vi "DPO_7K_NextState_Autoscale.vi"(5 "Upper Threshold":dbl, 6 "ATI?":bool, 7 "Lower Threshold":dbl, 8 "Offset":dbl, 9 "Current Vertical Scale":dbl, 10 "Waveform Maximum Value":dbl, 11 "Waveform Minumum Value":dbl) -> (3 "Autoscale States":T1)   [LabVIEW 2020]
uses:
  DPO_7K_Autoscale_States.ctl
panel:
  out "Minimum":dbl
  out "Maximum":dbl
  out "Acquisition warning":bool
  out "Increase vertical scale":bool
  out "Decrease vertical scale":bool
  out "Change Offset":bool
  out "Valid Acquisition, Exit":bool
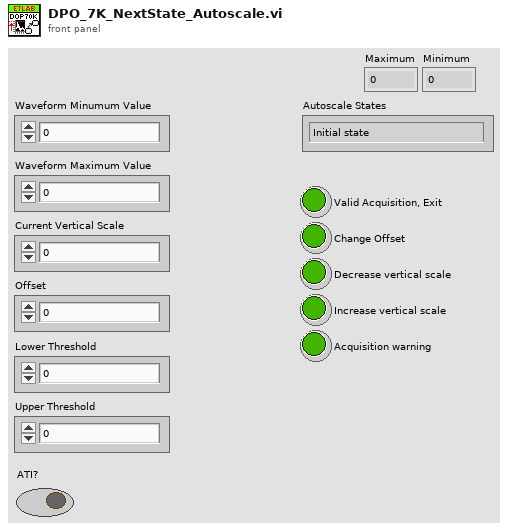
[diagram p1: front panel]
types:
  T1 = typedef "DPO_7K_Autoscale_States.ctl" = enum16{"Initial state", "Change offset", "Increase scale", "Decrease scale", "Acquisition warning", "General error", "Exit"}
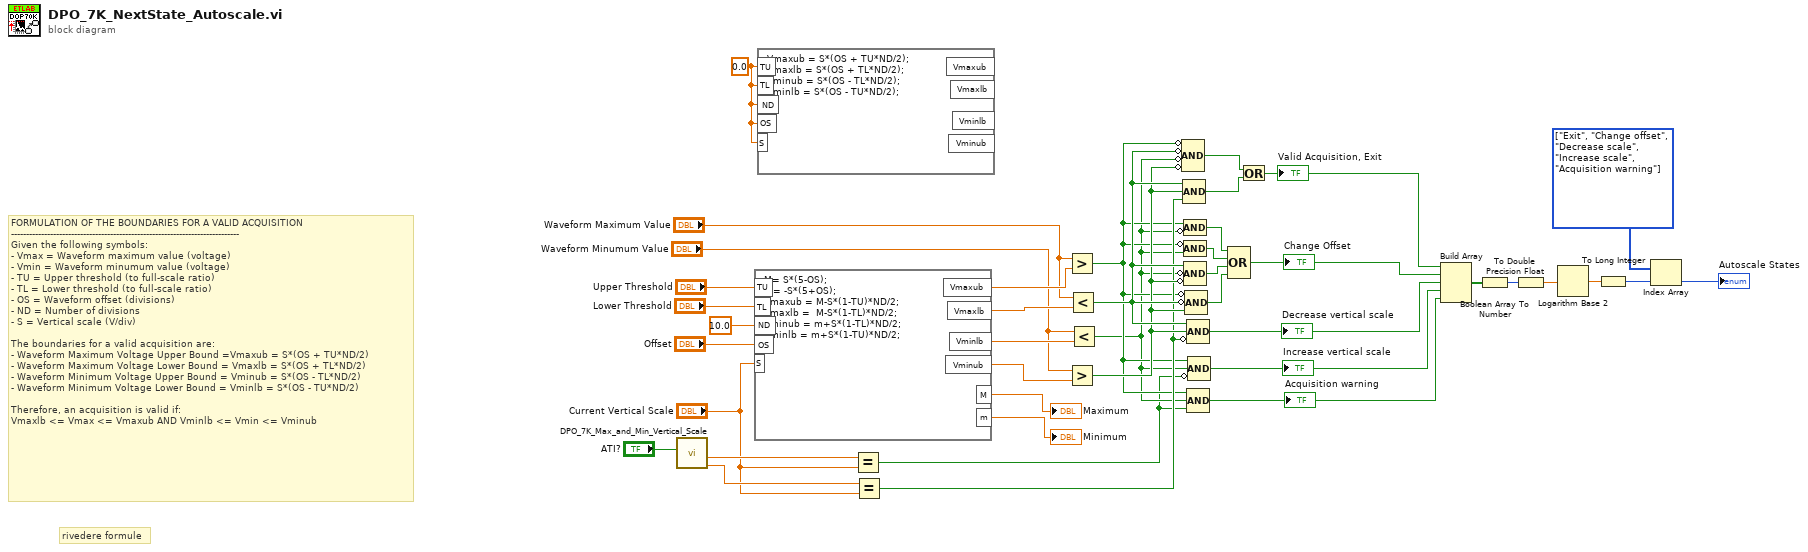
[diagram p0: block diagram]
diagram:
  w3 = 0.0 ("input variable")
  w5 = T1[] [enum."Exit", enum."Change offset", enum."Decrease scale", enum."Increase scale", enum."Acquisition warning"] items=["Initial state", "Change offset", "Increase scale", "Decrease scale", "Acquisition warning", "General error", "Exit"]
  # "rivedere formule"
  # "FORMULATION OF THE BOUNDARIES FOR A VALID ACQUISITION\n----------------------------------------------------------------------------\nGiven the following symbols:\n- Vmax = Waveform maximum value (voltage)\n- Vmin = Waveform minumum value (voltage)\n- TU = Upper threshold (to full-scale ratio)\n- TL = Lower threshold (to full-scale ratio)\n- OS = Waveform offset (divisions)\n- ND = Number of divisions\n- S = Vertical scale (V/div)\n\nThe boundaries for a valid acquisition are:\n- Waveform Maximum Voltage Upper Bound =Vmaxub = S*(OS + TU*ND/2)\n- Waveform Maximum Voltage Lower Bound = Vmaxlb = S*(OS + TL*ND/2)\n- Waveform Minimum Voltage Upper Bound = Vminub = S*(OS - TL*ND/2)\n- Waveform Minimum Voltage Lower Bound = Vminlb = S*(OS - TU*ND/2)\n\nTherefore, an acquisition is valid if:\nVmaxlb <= Vmax <= Vmaxub AND Vminlb <= Vmin <= Vminub"
  n1 = call "DPO_7K_Max_and_Min_Vertical_Scale.vi"("ATI?"="ATI?") -> ("Min"=w39:dbl, "Max"=w40:dbl)  [unwired: 9 in]
  n2 = formula code="M= S*(5-OS);\nm= -S*(5+OS);\nVmaxub = M-S*(1-TU)*ND/2;\nVmaxlb =  M-S*(1-TL)*ND/2;\nVminub = m+S*(1-TL)*ND/2;\nVminlb = m+S*(1-TU)*ND/2;"("TU"="Upper Threshold", "TL"="Lower Threshold", "ND"=10.0 ("input variable"), "OS"="Offset", "S"="Current Vertical Scale") -> ("Vmaxub"=w33:dbl, "Vminlb"=w31:dbl, "Vminub"=w30:dbl, "Vmaxlb"=w32:dbl, "M"=→"Maximum":dbl, "m"=→"Minimum":dbl)
  n3 = formula code="Vmaxub = S*(OS + TU*ND/2);\nVmaxlb = S*(OS + TL*ND/2);\nVminub = S*(OS - TL*ND/2);\nVminlb = S*(OS - TU*ND/2);"("TU"=w3, "TL"=w3, "ND"=w3, "OS"=w3, "S"=w3) -> ()  [unwired: 4 out]
  n4 = Equal?(x=w40, y="Current Vertical Scale") -> (x = y?=w16:bool)
  n5 = Equal?(x=w39, y="Current Vertical Scale") -> (x = y?=w19:bool)
  n6 = Greater?(x="Waveform Maximum Value", y=w33) -> (0:w18:bool)
  n7 = Greater?(x="Waveform Minumum Value", y=w30) -> (0:w20:bool)
  n8 = Less?(x="Waveform Maximum Value", y=w32) -> (x < y?=w21:bool)
  n9 = Less?(x="Waveform Minumum Value", y=w31) -> (x < y?=w17:bool)
  n10 = Compound Arithmetic op=AND(invert w18, invert w21, invert w17, invert w20) -> (w23:bool)
  n11 = Compound Arithmetic op=AND(w21, w20, w19) -> (w24:bool)
  n12 = Compound Arithmetic op=AND(w18, invert w17) -> (w29:bool)
  n13 = Compound Arithmetic op=AND(invert w18, w17) -> (w28:bool)
  n14 = Compound Arithmetic op=AND(w21, invert w17, invert w20) -> (w27:bool)
  n15 = Compound Arithmetic op=AND(invert w18, invert w21, w20) -> (w22:bool)
  n16 = Compound Arithmetic op=AND(w21, w20, invert w19) -> (w13:bool)
  "Decrease vertical scale" <- w13
  n17 = Compound Arithmetic op=AND(w18, w17, w16) -> (w11:bool)
  "Acquisition warning" <- w11
  n18 = Compound Arithmetic op=AND(w18, w17, invert w16) -> (w12:bool)
  "Increase vertical scale" <- w12
  n19 = Compound Arithmetic op=OR(w29, w28, w27, w22) -> (w14:bool)
  "Change Offset" <- w14
  n20 = Or(x=w23, y=w24) -> (x .or. y?=w15:bool)
  "Valid Acquisition, Exit" <- w15
  n21 = Build Array(w15, w14, w13, w12, w11) -> (w10:bool[])
  n22 = Boolean Array To Number(Boolean array=w10) -> (number=w9:u32)
  n23 = To Double Precision Float(number=w9) -> (double precision float=w8:dbl)
  n24 = Logarithm Base 2(1:w8) -> (0:w7:dbl)
  n25 = To Long Integer(number=w7) -> (32bit integer=w6:i32)
  n26 = Index Array(array=w5, index=w6) -> (element=→"Autoscale States":T1)
